vi "CCImageToDcmPopulateDatasetDicomTag.vi"(6 "dic in":refnum<k24>, 8 "error in (no error)":errorcluster, 9 "tagName":string, 10 "stringValue":string, 11 "Dataset in":refnum<k24>) -> (0 "error out":errorcluster, 2 "Dic out":refnum<k24>, 3 "Dataset out":refnum<k24>)   [LabVIEW 2013, in "main.lvlib" / "ClearCanvasLibrary.lvlib"]
uses:
  ClearCanvasLibrary.lvlib
  C:/Users/Simon/SkyDrive/LabView/2013/DM2020/DICOM/ClearCanvasNewBuild/ClearCanvas.Dicom.dll
  ClearCanvasNewBuild/ClearCanvas.Dicom.dll
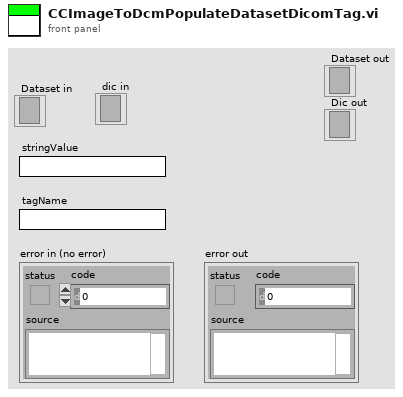
[diagram p1: front panel]
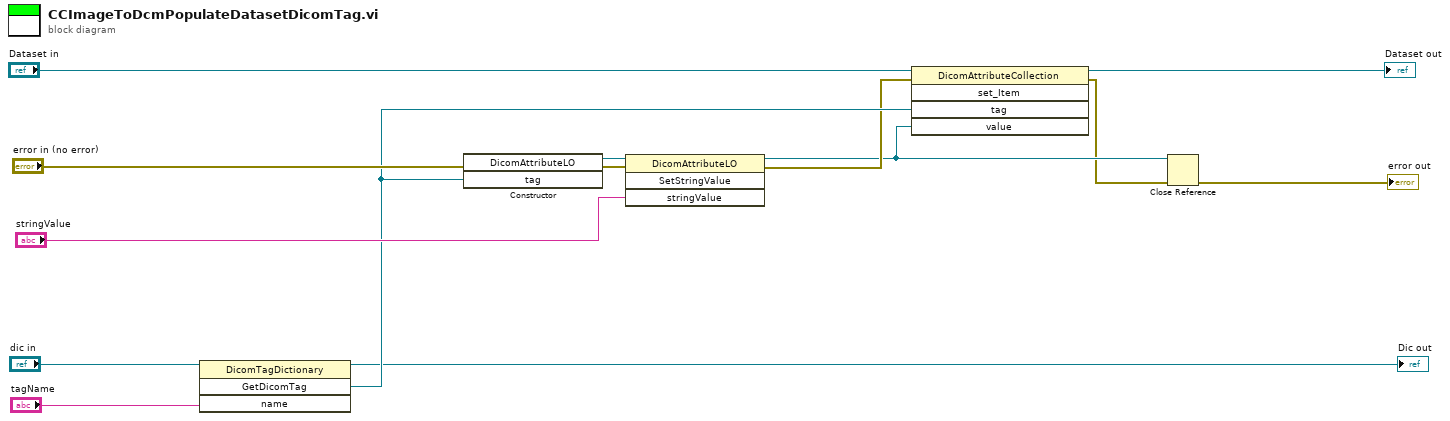
[diagram p0: block diagram]
diagram:
  n1 = invoke class="DicomTagDictionary" method="GetDicomTag"(reference="dic in", "name"="tagName") -> (reference out=→"Dic out":refnum<k24>, "GetDicomTag"=w10:refnum<k24>)  [unwired: 2 in, 2 out]
  n2 = constructor class="DicomAttributeLO"(error in="error in (no error)", "tag"=w10) -> (reference out=w2:refnum<k24>, error out=w1:errorcluster)  [unwired: 2 in, 2 out]
  n3 = invoke class="DicomAttributeLO" method="SetStringValue"(reference=w2, error in=w1, "stringValue"="stringValue") -> (reference out=w5:refnum<k24>, error out=w9:errorcluster)  [unwired: 1 in, 2 out]
  n4 = invoke class="DicomAttributeCollection" method="set_Item"(reference="Dataset in", error in=w9, "tag"=w10, "value"=w5) -> (reference out=→"Dataset out":refnum<k24>, error out=w4:errorcluster)  [unwired: 1 in, 3 out]
  n5 = Close Reference(reference=w5, error in (no error)=w4) -> (error out=→"error out":errorcluster)
